vi "ConvertClients.vi"(11 "ClientList":T1) -> (3 "ClientListArray":string[][](array[string]))   [LabVIEW 2017, in "Server.lvlib"]
doc: "Converts Array of Clusters \"Client List.ctl\" to String Array for displaying."
uses:
  Server.lvlib
  TypeDefs/ClientList.ctl
  TypeDefs/ClientData.ctl
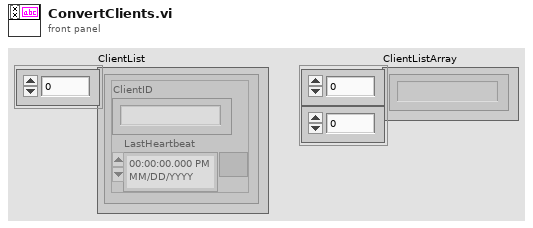
[diagram p1: front panel]
types:
  T1 = typedef "Server.lvlib/ClientList.ctl" = T2[]
  T2 = typedef "Server.lvlib/ClientData.ctl" = cluster{"ClientID":string, "LastHeartbeat":timestamp}
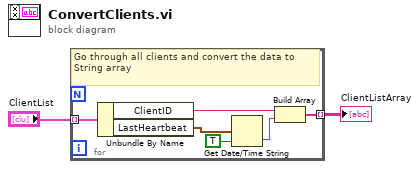
[diagram p0: block diagram]
diagram:
  n1 = for {
    tunnel: "ClientList" -> [w8] mode=indexing
    tunnel: [w4] -> w2 mode=indexing
    # "Go through all clients and convert the data to String array"
    n2 = Unbundle By Name(w8) -> ("ClientID"=w5:string, "LastHeartbeat"=w7:timestamp)
    n3 = Get Date/Time String(seconds (now)=w7, want seconds? (F)=TRUE) -> (time string=w6:string)  [unwired: 1 in, 1 out]
    n4 = Build Array(w5, w6) -> (w4:string[])
  }
  "ClientListArray" <- w2
